vi "Lab10_v2_template.vi"() -> ()   [LabVIEW 2020]
doc: "This example demonstrates how to continuously re-generate analog output data from a buffer in your computer's memory.\n\nRefer to your device documentation for pinouts and hardware capabilities."
uses:
  <vilib>/DAQmx/write.llb/DAQmx Write (Analog Wfm 1Chan NSamp).vi
  <vilib>/DAQmx/read.llb/DAQmx Read (Analog 1D Wfm NChan NSamp).vi
  <vilib>/DAQmx/create/channels.llb/DAQmx Create Channel (AO-Voltage-Basic).vi
  <vilib>/DAQmx/configure/timing.llb/DAQmx Timing (Sample Clock).vi
  <vilib>/DAQmx/miscellaneous.llb/DAQmx Fill In Error Info.vi
  <vilib>/DAQmx/create/channels.llb/DAQmx Create Channel (AI-Voltage-Basic).vi
  <vilib>/measure/NI_MABase.lvlib
panel:
  in  "Amplitude":dbl=1.0 format="%0.2p"
  in  "Frequency":dbl=10.0 format="%0.2p"
  in  "Waveform Type":u16(ring) items=["Sine Wave", "Triangle Wave", "Square Wave", "Sawtooth Wave"]
  in  "Input Channel 2":tag="Dev6/ai1"
  in  "Number of samples":i32=1000
  out "Input Voltage":waveform(dbl)[](graph)=[{"t0"=timestamp(3702416907.610318 s since 1904-01-01), "dt"=9.999999999999999e-05, "Y"=array[1000 elements], "attributes"=variant("NI_ChannelName"=variant(string "Dev6/ai0"), "NI_UnitDescription"=variant(string "Volts"))}, {"t0"=timestamp(3702416907.610332 s since 1904-01-01), "dt"=9.999999999999999e-05, "Y"=array[1000 elements], "attributes"=variant("NI_ChannelName"=variant(string "Dev6/ai1"), "NI_UnitDescription"=variant(string "Volts"))}]
  in  "Input Channel 1":tag="Dev6/ai0"
  in  "Min Input Voltage":dbl=-10.0
  in  "Max Input Voltage":dbl=10.0
  in  "Output sample rate":dbl=10000.0 format="%0.2f"
  out "Output Voltage":waveform(dbl)(graph)={"t0"=timestamp(0 s since 1904-01-01), "dt"=0.0001, "Y"=array[1000 elements]}
  in  "Max Voltage":dbl=10.0
  in  "Min Voltage":dbl=-10.0
  in  "Output Channel":tag="Dev6/ao0"
  # "Output Channel Settings"
  # "Output voltage"
  # "Input voltage"
  # "Input Channel Settings"
  # "Waveform Settings"
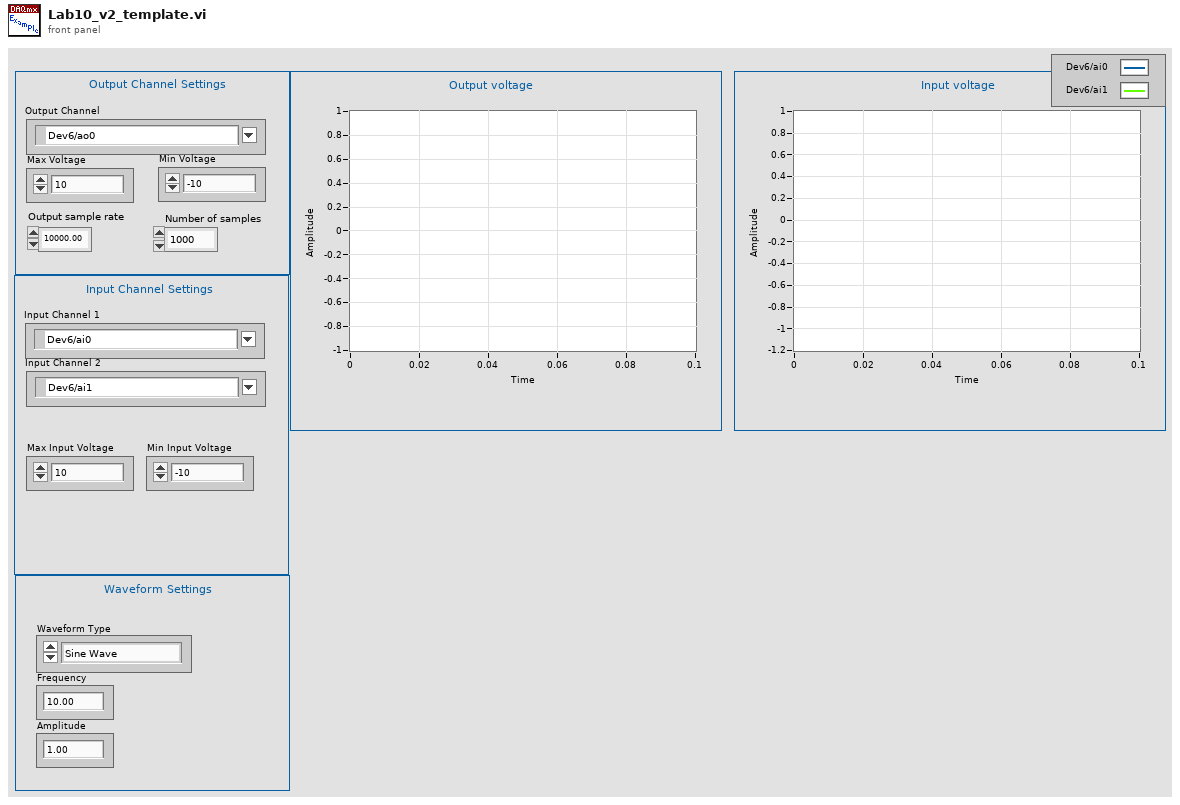
[diagram p1: front panel]
types:
  T1 = cluster{"Output sample rate":dbl, "Number of samples":i32}
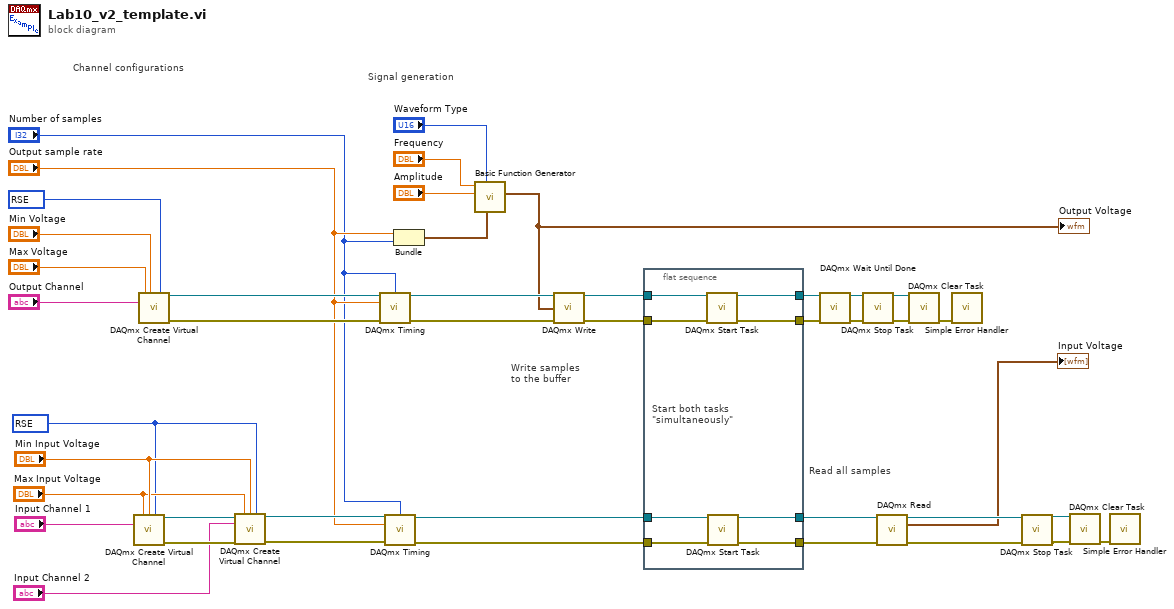
[diagram p0: block diagram]
diagram:
  w12 = 10083 items=["Default"=-1, "RSE"=10083, "NRSE"=10078, "Differential"=10106, "Pseudodifferential"=12529] ("input terminal configuration")
  w32 = 10083 items=["Default"=-1, "RSE"=10083, "NRSE"=10078, "Differential"=10106, "Pseudodifferential"=12529] ("input terminal configuration")
  # "Read all samples"
  # "Write samples\nto the buffer"
  # "Signal generation"
  # "Channel configurations"
  n1 = call-poly <vilib>:"DAQmx Create Virtual Channel.vi"("maximum value"="Max Input Voltage", "minimum value"="Min Input Voltage", "input terminal configuration"=w12, "physical channels"="Input Channel 1") -> ("task out"=w22:refnum<k21>, "error out"=w23:errorcluster)  [unwired: 10 in]
  n2 = call-poly <vilib>:"DAQmx Create Virtual Channel.vi"("maximum value"="Max Voltage", "minimum value"="Min Voltage", "output terminal configuration"=w32, "physical channels"="Output Channel") -> ("task out"=w36:refnum<k21>, "error out"=w37:errorcluster)  [unwired: 10 in]
  n3 = call-poly <vilib>:"DAQmx Create Virtual Channel.vi"("task in"=w22, "maximum value"="Max Input Voltage", "minimum value"="Min Input Voltage", "input terminal configuration"=w12, "physical channels"="Input Channel 2", "error in"=w23) -> ("task out"=w21:refnum<k21>, "error out"=w20:errorcluster)  [unwired: 8 in]
  n4 = call-poly <vilib>:"DAQmx Timing.vi"("task/channels in"=w36, "samples per channel"="Number of samples", "rate"="Output sample rate", "error in"=w37) -> ("task out"=w29:refnum<k21>, "error out"=w10:errorcluster)  [unwired: 10 in]
  n5 = call-poly <vilib>:"DAQmx Timing.vi"("task/channels in"=w21, "samples per channel"="Number of samples", "rate"="Output sample rate", "error in"=w20) -> ("task out"=w28:refnum<k21>, "error out"=w27:errorcluster)  [unwired: 10 in]
  n6 = Bundle "Bundle"("Output sample rate"="Output sample rate", "Number of samples"="Number of samples") -> (w11:T1)  [unwired: 1 in]
  n7 = call <vilib>:"Basic Function Generator.vi"("sampling info"=w11, "signal type"="Waveform Type", "amplitude"="Amplitude", "frequency"="Frequency") -> ("signal out"=w24:waveform(dbl))  [unwired: 5 in, 2 out]
  "Output Voltage" <- w24
  n8 = call-poly <vilib>:"DAQmx Write.vi"("task/channels in"=w29, "data"=w24, "error in"=w10) -> ("task out"=w26:refnum<k21>, "error out"=w25:errorcluster)  [unwired: 10 in, 1 out]
  n9 = flat-sequence {
    tunnel: w28 -> [w51]
    tunnel: w27 -> [w50]
    tunnel: [w49] -> w6
    tunnel: [w45] -> w5
    tunnel: w26 -> [w48]
    tunnel: w25 -> [w44]
    tunnel: [w47] -> w3
    tunnel: [w46] -> w4
    frame #0 {
      # "Start both tasks\n\"simultaneously\""
      n10 = call <vilib>:"DAQmx Start Task.vi"("task/channels in"=w48, "error in"=w44) -> ("task out"=w46:refnum<k21>, "error out"=w47:errorcluster)  [unwired: 12 in]
      n11 = call <vilib>:"DAQmx Start Task.vi"("task/channels in"=w51, "error in"=w50) -> ("task out"=w49:refnum<k21>, "error out"=w45:errorcluster)  [unwired: 12 in]
    }
  }
  n12 = call <vilib>:"DAQmx Wait Until Done.vi"("task/channels in"=w4, "error in"=w3) -> ("task out"=w2:refnum<k21>, "error out"=w1:errorcluster)  [unwired: 12 in]
  n13 = call <vilib>:"DAQmx Stop Task.vi"("task/channels in"=w2, "error in"=w1) -> ("task out"=w39:refnum<k21>, "error out"=w38:errorcluster)  [unwired: 12 in]
  n14 = call-poly <vilib>:"DAQmx Read.vi"("task/channels in"=w6, "error in"=w5) -> ("task out"=w30:refnum<k21>, "data"=→"Input Voltage":waveform(dbl)[], "error out"=w31:errorcluster)  [unwired: 11 in]
  n15 = call <vilib>:"DAQmx Clear Task.vi"("task in"=w39, "error in"=w38) -> ("error out"=w43:errorcluster)  [unwired: 13 in]
  n16 = call <vilib>:"Simple Error Handler.vi"("error in (no error)"=w43) -> ()  [unwired: 4 in, 5 out]
  n17 = call <vilib>:"DAQmx Stop Task.vi"("task/channels in"=w30, "error in"=w31) -> ("task out"=w34:refnum<k21>, "error out"=w35:errorcluster)  [unwired: 12 in]
  n18 = call <vilib>:"DAQmx Clear Task.vi"("task in"=w34, "error in"=w35) -> ("error out"=w33:errorcluster)  [unwired: 13 in]
  n19 = call <vilib>:"Simple Error Handler.vi"("error in (no error)"=w33) -> ()  [unwired: 4 in, 5 out]
